vi "Sequence.vi"() -> (3 "Cancelled?":bool caption="キャンセルされた?")   [LabVIEW 2017]
doc: "イベント処理を使用するダイアログボックスを作成するのにこのテンプレートを使用します。"
uses:
  controls/Param_static_AF.ctl
panel:
  out "配列":string[](array[string])
  in  "staticAF parameters":T1={"Axis"=0, "Peak field (Oe) "=2, "Ramp rate"=3, "Hold time (ms)"=0} {"Ramp rate" min=1 max=9 step=2; "Peak field (Oe)" min=2 max=1200; "Axis" items=["X", "Y", "Z"]}
  in  "static AF":bool
  out "Sequence":string
  in  "Load":bool
  in  "Save as":bool
  in  "Cancel":bool caption="キャンセル"
  in  "OK":bool
  # "Add treatment"
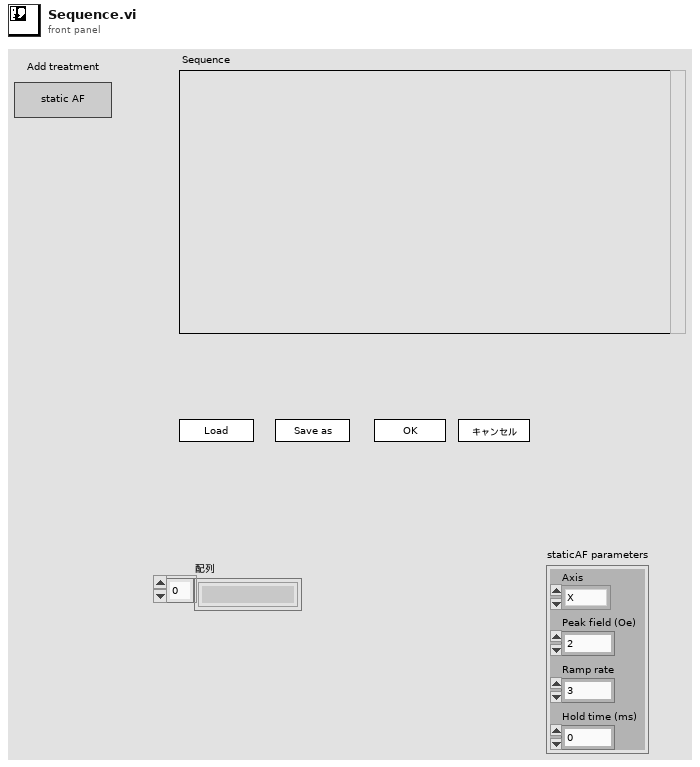
[diagram p1: front panel]
types:
  T1 = typedef "Param_static_AF.ctl" = cluster{"Axis":u16, "Peak field (Oe) ":u16, "Ramp rate":u8, "Hold time (ms)":u16}
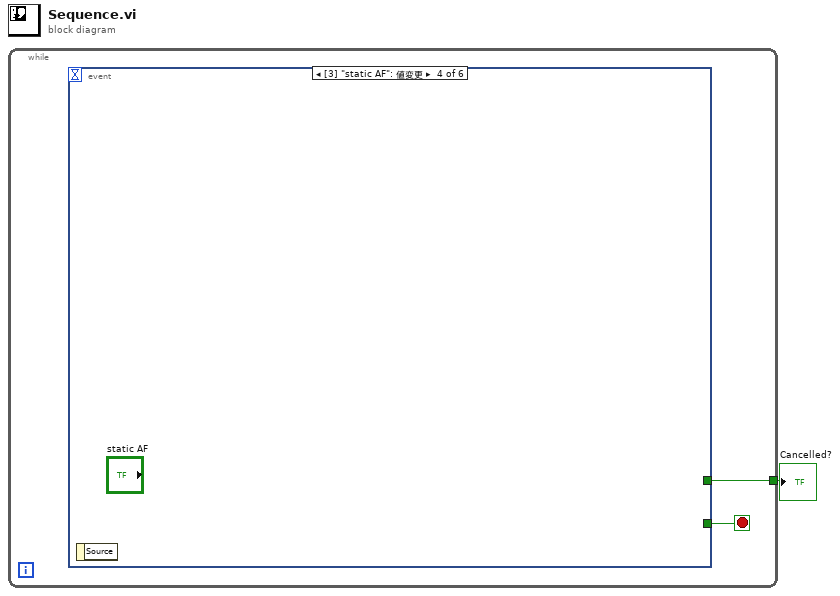
[diagram p0: block diagram]
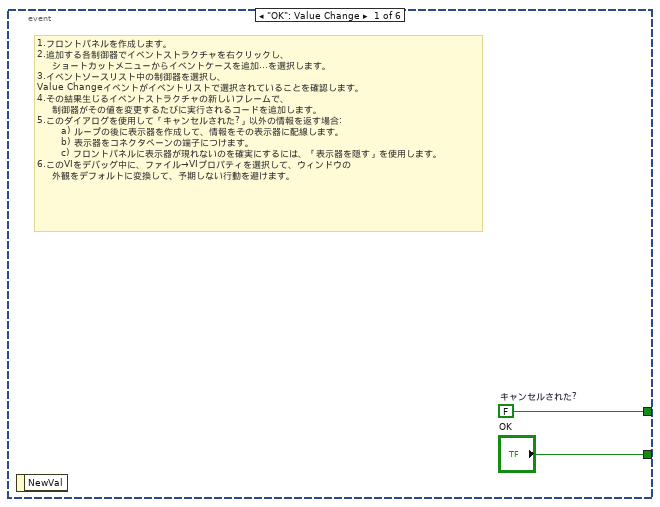
[diagram p2: hidden frame]
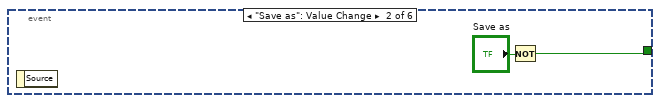
[diagram p3: hidden frame]
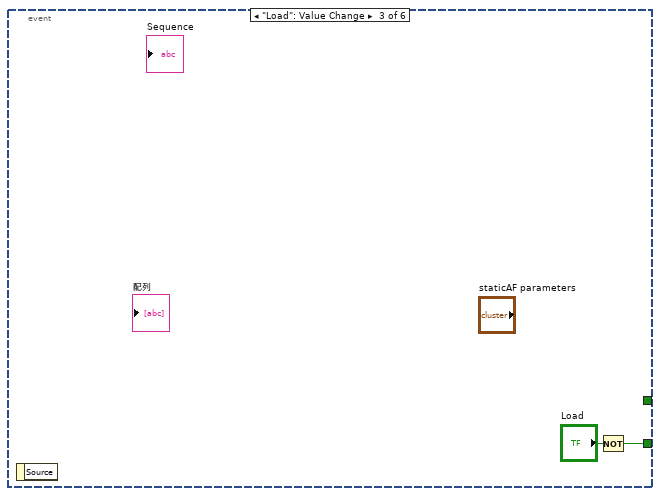
[diagram p4: hidden frame]
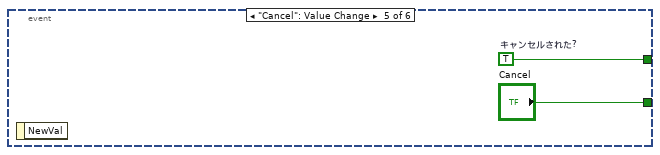
[diagram p5: hidden frame]
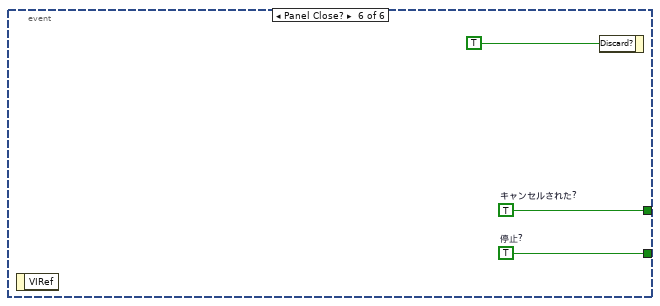
[diagram p6: hidden frame]
diagram:
  n1 = while {
    tunnel: [w2] -> w1
    stop <- w3 stop-if-true
    n2 = event shown="[3] \"static AF\": 値変更" {
      selector: _ -> [_ _ _ _ _ _]
      dyn-events: _ -> [_ _ _ _ _ _]
      timeout: _ -> [_ _ _ _ _ _]
      tunnel: ["OK" w6 w8 _ "Cancel" w13] -> w3
      tunnel: [w5 _ _ _ w11 w12] -> w2
      event "OK": Value Change {
        w5 = FALSE  # キャンセルされた?
        # "1.フロントパネルを作成します。\n2.追加する各制御器でイベントストラクチャを右クリックし、\n     ショートカットメニューからイベントケースを追加...を選択します。\n3.イベントソースリスト中の制御器を選択し、\nValue Changeイベントがイベントリストで選択されていることを確認します。\n4.その結果生じるイベントストラクチャの新しいフレームで、\n     制御器がその値を変更するたびに実行されるコードを追加します。\n5.このダイアログを使用して「キャンセルされた?」以外の情報を返す場合:\n        a) ループの後に表示器を作成して、情報をその表示器に配線します。\n        b) 表示器をコネクタペーンの端子につけます。\n        c) フロントパネルに表示器が現れないのを確実にするには、「表示器を隠す」を使用します。\n6.このVIをデバッグ中に、ファイル→VIプロパティを選択して、ウィンドウの\n     外観をデフォルトに変換して、予期しない行動を避けます。"
        n3 = event-data() -> ()  [unwired: 1 in, 1 out]
      }
      event "Save as": Value Change {
        n4 = event-data() -> ()  [unwired: 1 in, 1 out]
        n5 = Not(x="Save as") -> (.not. x?=w6:bool)
      }
      event "Load": Value Change {
        n6 = event-data() -> ()  [unwired: 1 in, 1 out]
        n7 = Not(x="Load") -> (.not. x?=w8:bool)
      }
      event "static AF": Value Change {
        n8 = event-data() -> ()  [unwired: 1 in, 1 out]
      }
      event "Cancel": Value Change {
        w11 = TRUE  # キャンセルされた?
        n9 = event-data() -> ()  [unwired: 1 in, 1 out]
      }
      event Panel Close? {
        w12 = TRUE  # キャンセルされた?
        w13 = TRUE  # 停止?
        n10 = event-data() -> ()  [unwired: 1 in, 1 out]
        n11 = event-data("Discard?"=TRUE) -> ()  [unwired: 1 in, 1 out]
      }
    }
  }
  "Cancelled?" <- w1
